vi "GetMFCFlows.vi"(1 "Indices":i32[](array[numeric])) -> (0 "Flows":dbl[](array[numeric]))   [LabVIEW 2011]
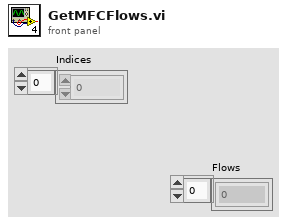
[diagram p1: front panel]
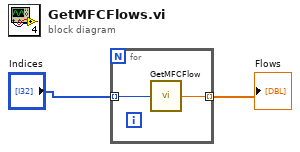
[diagram p0: block diagram]
diagram:
  n1 = for {
    tunnel: "Indices" -> [w4] mode=indexing
    tunnel: [w3] -> w1 mode=indexing
    n2 = call "GetMFCFlow.vi"("MFC ID Number"=w4) -> ("Flow"=w3:dbl)
  }
  "Flows" <- w1
